vi "Post-Build Custom Action.vi"() -> (0 "error out":errorcluster)   [LabVIEW 2021]
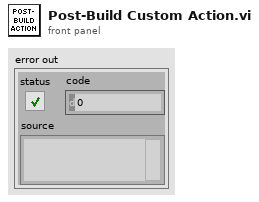
[diagram p1: front panel]
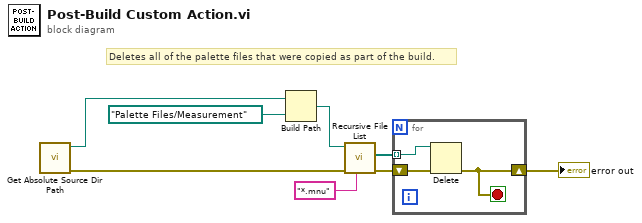
[diagram p0: block diagram]
diagram:
  # "Deletes all of the palette files that were copied as part of the build."
  n1 = call "Get Absolute Source Dir Path.vi"() -> ("error out"=w5:errorcluster, "source dir"=w3:path)  [unwired: 10 in]
  n2 = Build Path(base path=w3, name or relative path=path "Palette Files/Measurement") -> (appended path=w6:path)
  n3 = call <vilib>:"Recursive File List.vi"("pattern"="*.mnu", "error in (no error)"=w5, "Folder Path"=w6) -> ("error out"=w8:errorcluster, "All Files in Dir"=w4:path[])  [unwired: 4 in, 3 out]
  n4 = for {
    tunnel: w4 -> [w11] mode=indexing
    shift-right: [w9] -> w7
    shift-left: w8 -> [w10]
    stop <- w9 stop-if-true
    n5 = Delete(path (use dialog)=w11, error in=w10) -> (error out=w9:errorcluster)  [unwired: 3 in, 2 out]
  }
  "error out" <- w7
